vi "Set Speed.vi"(8 "error in (no error)":errorcluster, 10 "Pump %":sgl, 11 "ASIA Pump C Settings in":T1) -> (0 "error out":errorcluster, 1 "Connection Error":bool, 3 "ASIA Pump C Settings out":T1)   [LabVIEW 2018, in "ASIA Pump.lvlib"]
uses:
  ASIA Pump.lvlib
  Pump Settings.ctl
panel:
  out "path out":path
  out "Status Connection Error":bool
  out "Task Completed":bool
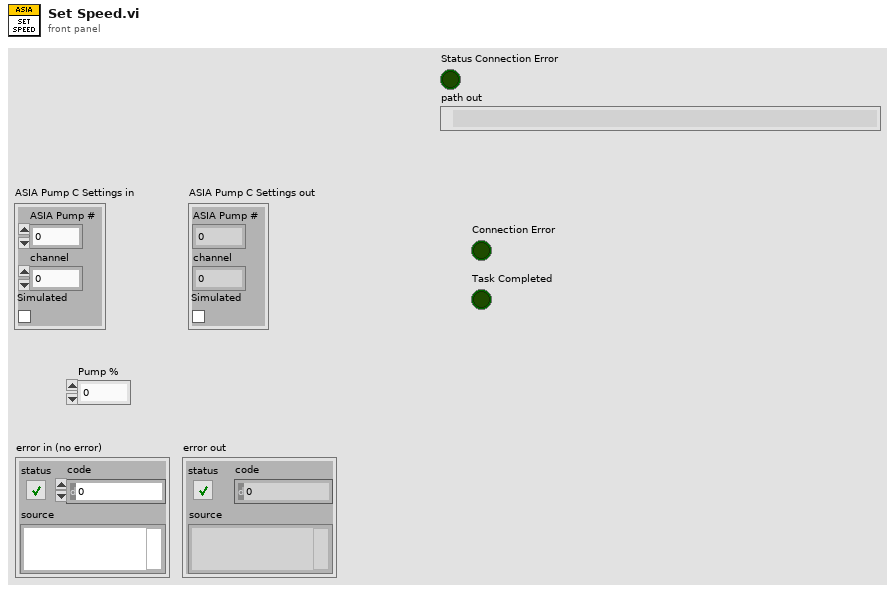
[diagram p1: front panel]
types:
  T1 = typedef "ASIA Pump.lvlib/Pump Settings.ctl" = cluster{"ASIA Pump #":i32, "channel":i32, "Simulated":bool}
  T2 = enum16{"Error", "Uninitialised", "Initialising", "Idle", "Filling", "Full", "Emptying", "Empty", "Pumping", "Default"}
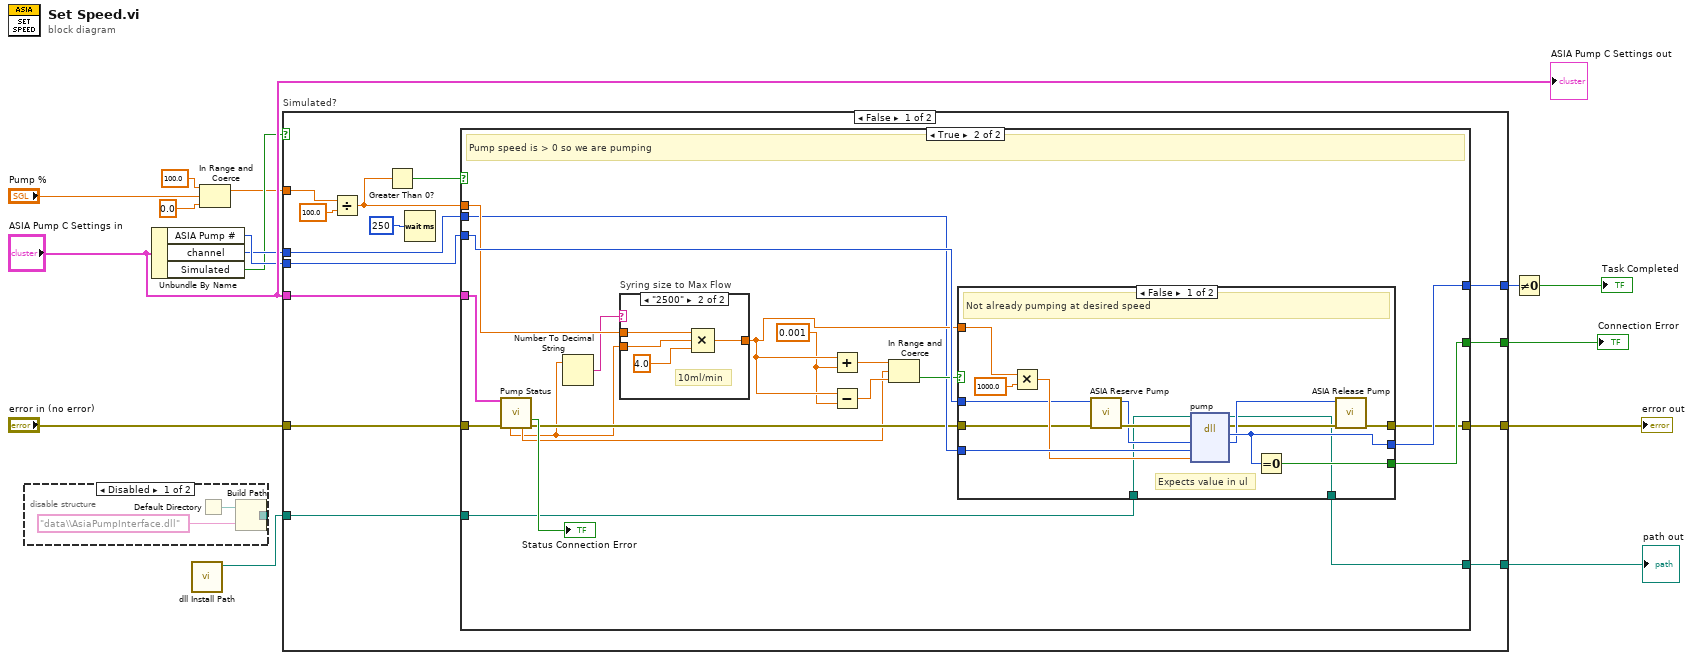
[diagram p0: block diagram]
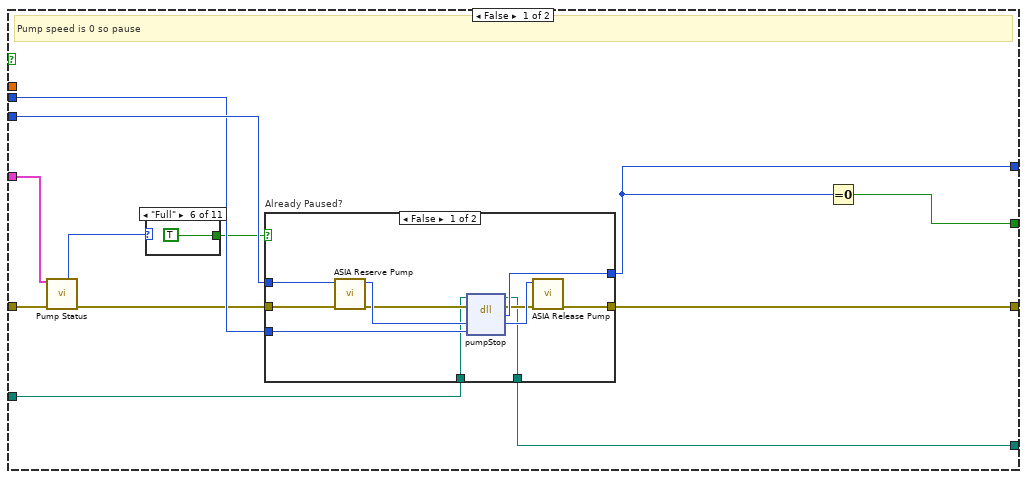
[diagram p3: hidden frame]
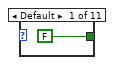
[diagram p4: hidden frame]
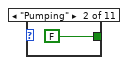
[diagram p5: hidden frame]
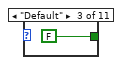
[diagram p6: hidden frame]
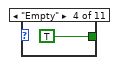
[diagram p7: hidden frame]
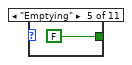
[diagram p8: hidden frame]
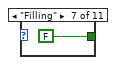
[diagram p9: hidden frame]
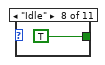
[diagram p10: hidden frame]
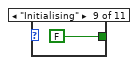
[diagram p11: hidden frame]
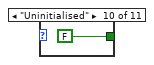
[diagram p12: hidden frame]
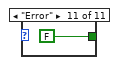
[diagram p13: hidden frame]
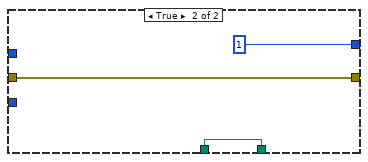
[diagram p14: hidden frame]
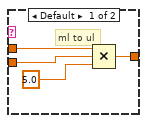
[diagram p15: hidden frame]
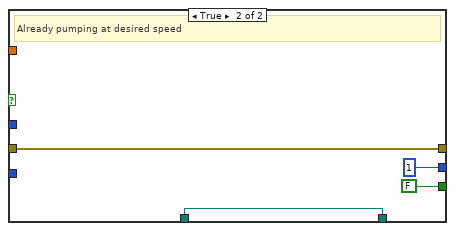
[diagram p16: hidden frame]
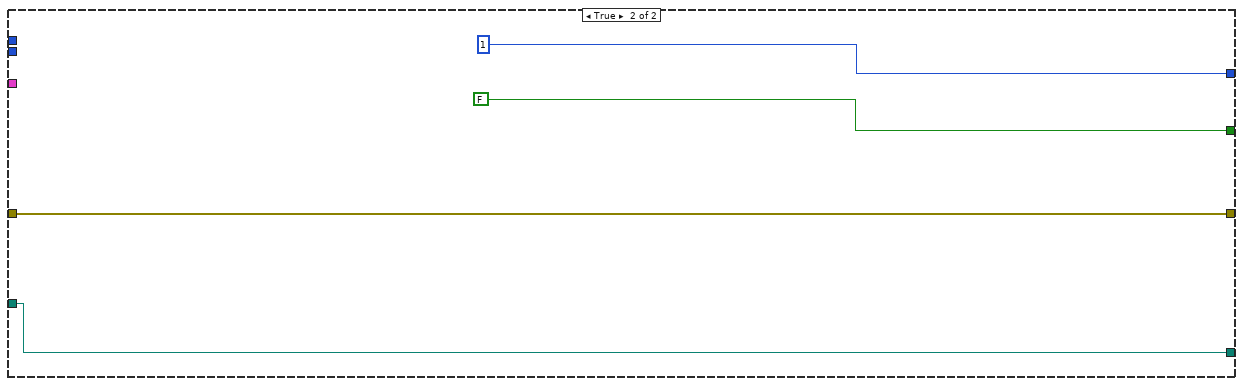
[diagram p17: hidden frame]
diagram:
  n1 = disable-structure shown="Disabled" {
    disable-tunnel: [w16 _] -> _
    frame Disabled {
      n2 = Default Directory() -> (w17:path)
      n3 = Build Path(base path=w17, name or relative path="data\\AsiaPumpInterface.dll") -> (appended path=w16:path)
    }
    frame Enabled {
    }
  }
  n4 = Unbundle By Name("ASIA Pump C Settings in") -> ("ASIA Pump #"=w10:i32, "channel"=w9:i32, "Simulated"=w7:bool)
  n5 = call "dll Install Path.vi"() -> ("system directory"=w1:path)  [unwired: 11 in]
  n6 = In Range and Coerce(upper limit=100.0, x="Pump %", lower limit=0.0) -> (coerced(x)=w3:dbl)  [unwired: 1 out]
  n7 = case "Simulated?" shown="False" w7 {
    tunnel: [w32 w120] -> w14
    tunnel: "ASIA Pump C Settings in" -> [w31 _]
    tunnel: "error in (no error)" -> [w30 w120]
    tunnel: w10 -> [w29 _]
    tunnel: w9 -> [w28 _]
    tunnel: [w27 FALSE ("Connection Error")] -> w11
    tunnel: [w26 1 ("Bool")] -> w8
    tunnel: w3 -> [w24 _]
    tunnel: [w20 w117] -> w2
    tunnel: w1 -> [w19 w117]
    frame False {
      n8 = Divide(x=w24, y=sgl 100.0) -> (x/y=w23:dbl)
      n9 = Greater Than 0?(x=w23) -> (x > 0?=w22:bool)
      n10 = Wait (ms)(milliseconds to wait=u32 250) -> ()  [unwired: 1 out]
      n11 = case shown="True" w22 {
        tunnel: [w42 w79] -> w32
        tunnel: w29 -> [w44 w89]
        tunnel: w28 -> [w43 w78]
        tunnel: w23 -> [_ w86]
        tunnel: [w40 w88] -> w27
        tunnel: [w39 w87] -> w26
        tunnel: w30 -> [w36 w77]
        tunnel: w31 -> [w38 w76]
        tunnel: w19 -> [w34 w71]
        tunnel: [w33 w70] -> w20
        frame False {
          # "Pump speed is 0 so pause"
          n12 = call "Pump Status.vi"("ASIA Pump C Settings in"=w38, "error in (no error)"=w36) -> ("PumpStatusCode"=w37:T2, "error out"=w35:errorcluster)  [unwired: 5 in, 7 out]
          n13 = case shown="\"Full\"" w37 {
            tunnel: [FALSE FALSE FALSE TRUE FALSE TRUE FALSE TRUE FALSE FALSE FALSE] -> w41
            frame Default {
            }
            frame "Pumping" {
            }
            frame "Default" {
            }
            frame "Empty" {
            }
            frame "Emptying" {
            }
            frame "Full" {
            }
            frame "Filling" {
            }
            frame "Idle" {
            }
            frame "Initialising" {
            }
            frame "Uninitialised" {
            }
            frame "Error" {
            }
          }
          n14 = case "Already Paused?" shown="False" w41 {
            tunnel: w44 -> [w64 _]
            tunnel: w43 -> [w66 _]
            tunnel: [w65 1 ("Bool")] -> w39
            tunnel: [w58 w69] -> w42
            tunnel: w35 -> [w61 w69]
            tunnel: w34 -> [w57 w67]
            tunnel: [w56 w67] -> w33
            frame False {
              n15 = call "ASIA Reserve Pump.vi"("error in (no error)"=w61, "ASIA Pump # In"=w64) -> ("error out"=w60:errorcluster, "ASIA Pump # Out"=w63:i32)  [unwired: 8 in]
              n16 = dll-call lib="C:/Program Files (x86)/Pfizer/FAST/data/AsiaPumpInterface.dll" fn="pumpStop"(path in=w57, error in=w60, "pumpNum"=w63, "channel"=w66) -> (path out=w56:path, error out=w59:errorcluster, "Bool"=w65:u8, "pumpNum"=w62:u32)  [unwired: 2 in]
              n17 = call "ASIA Release Pump.vi"("error in (no error)"=w59, "pumpNum"=w62) -> ("error out"=w58:errorcluster)  [unwired: 8 in, 1 out]
            }
            frame True {
            }
          }
          n18 = Equal To 0?(x=w39) -> (x = 0?=w40:bool)
        }
        frame True {
          w82 = 0.001 ("y")
          # "Pump speed is > 0 so we are pumping"
          n19 = call "Pump Status.vi"("ASIA Pump C Settings in"=w76, "error in (no error)"=w77) -> ("Connection Error"=→"Status Connection Error":bool, "syringeSize (ml)"=w72:sgl, "pumpRate"=w73:dbl, "error out"=w74:errorcluster)  [unwired: 5 in, 5 out]
          n20 = Number To Decimal String(number=w72) -> (decimal integer string=w85:string)  [unwired: 1 in]
          n21 = case "Syring size to Max Flow" shown="\"2500\"" w85 {
            tunnel: w86 -> [w91 w97]
            tunnel: [w90 w94] -> w83
            tunnel: w72 -> [w92 w96]
            frame Default {
              # "ml to ul"
              n22 = Compound Arithmetic op=MULTIPLY(w91, w92, 5.0 ("y")) -> (w90:dbl)
            }
            frame "2500" {
              # "10ml/min"
              n23 = Compound Arithmetic op=MULTIPLY(w97, w96, sgl 4.0 ("y")) -> (w94:dbl)
            }
          }
          n24 = Add(x=w83, y=w82) -> (x+y=w81:dbl)
          n25 = Subtract(x=w83, y=w82) -> (x-y=w80:dbl)
          n26 = In Range and Coerce(upper limit=w81, x=w73, lower limit=w80) -> (In Range?=w84:bool)  [unwired: 1 out]
          n27 = case shown="False" w84 {
            tunnel: w89 -> [w104 _]
            tunnel: w78 -> [w112 _]
            tunnel: w83 -> [w108 _]
            tunnel: [w111 FALSE] -> w88
            tunnel: w74 -> [w106 w114]
            tunnel: [w110 u8 1 ("Bool")] -> w87
            tunnel: [w100 w114] -> w79
            tunnel: w71 -> [w99 w113]
            tunnel: [w98 w113] -> w70
            frame False {
              # "Expects value in ul"
              # "Not already pumping at desired speed"
              n28 = Multiply(x=w108, y=1000.0) -> (x*y=w107:dbl)
              n29 = call "ASIA Reserve Pump.vi"("error in (no error)"=w106, "ASIA Pump # In"=w104) -> ("error out"=w105:errorcluster, "ASIA Pump # Out"=w103:i32)  [unwired: 8 in]
              n30 = dll-call lib="C:/Program Files (x86)/Pfizer/FAST/data/AsiaPumpInterface.dll" fn="pump"(path in=w99, error in=w105, "pumpNum"=w103, "channel"=w112, "rate"=w107) -> (path out=w98:path, error out=w101:errorcluster, "Bool"=w110:u8, "pumpNum"=w102:u32)  [unwired: 3 in]
              n31 = Equal To 0?(x=w110) -> (x = 0?=w111:bool)
              n32 = call "ASIA Release Pump.vi"("error in (no error)"=w101, "pumpNum"=w102) -> ("error out"=w100:errorcluster)  [unwired: 8 in, 1 out]
            }
            frame True {
              # "Already pumping at desired speed"
            }
          }
        }
      }
    }
    frame True {
    }
  }
  "Connection Error" <- w11
  "error out" <- w14
  "path out" <- w2
  n33 = Not Equal To 0?(x=w8) -> (x != 0?=→"Task Completed":bool)
  "ASIA Pump C Settings out" <- "ASIA Pump C Settings in"
